vi "2. Color Classification.vi"() -> ()   [LabVIEW 2019]
doc: "c 2020 ReMiSYS All rights reserved."
panel:
  out "Colors 2":string[](array[string])
  out "Colors":string[](array[string])
  out "appended path":path
  out "Input Image":T1(plugin-control)
  in  "Stop (F)":bool caption="Stop"
  in  "Loop Delay (ms)":u32(slide)=1000 scale=0.0..1500.0
  # "c 2020 ReMiSYS All rights reserved."
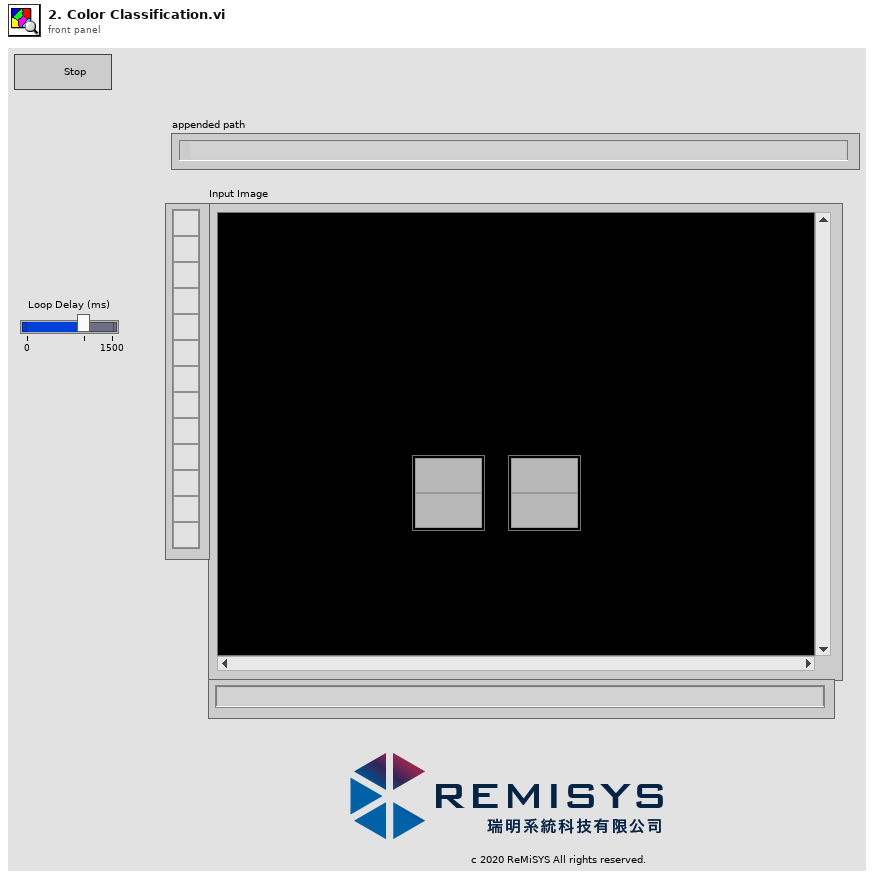
[diagram p1: front panel]
types:
  T1 = typedef "IMAQ Image.ctl" = refnum<image>
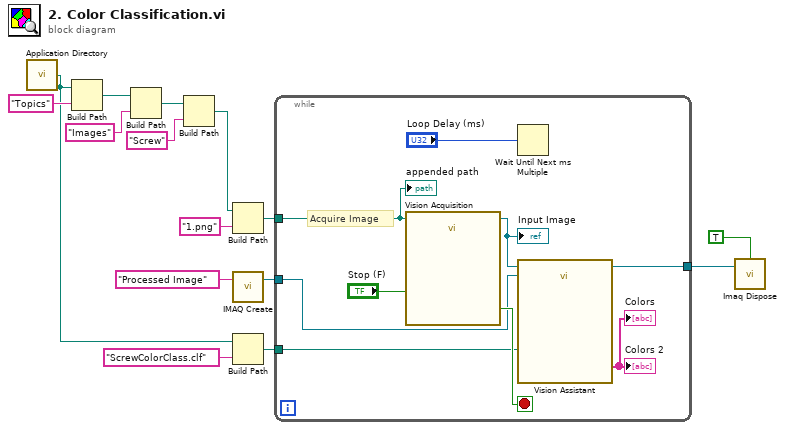
[diagram p0: block diagram]
diagram:
  n1 = call <vilib>:"Application Directory.vi"() -> ("Application Directory"=w1:path)
  n2 = Build Path(base path=w1, name or relative path="Topics") -> (appended path=w12:path)
  n3 = Build Path(base path=w12, name or relative path="Images") -> (appended path=w4:path)
  n4 = Build Path(base path=w4, name or relative path="Screw") -> (appended path=w5:path)
  n5 = Build Path(base path=w5, name or relative path="1.png") -> (appended path=w9:path)
  n6 = call "IMAQ Create"("Image Name"="Processed Image") -> ("New Image"=w15:T1)  [unwired: 3 in, 2 out]
  n7 = Build Path(base path=w1, name or relative path="ScrewColorClass.clf") -> (appended path=w2:path)
  n8 = while {
    tunnel: w15 -> [w20]
    tunnel: w9 -> [w21]
    tunnel: [w18] -> w8
    tunnel: w2 -> [w17]
    stop <- w24 stop-if-true
    # "Acquire Image"
    n9 = call "Vision Acquisition"("Image Path"=w21, "Stop (F)"="Stop (F)") -> ("Image Out"=w19:T1, "Stopped"=w24:bool)  [unwired: 1 in, 23 out]
    "Input Image" <- w19
    n10 = Wait Until Next ms Multiple(millisecond multiple="Loop Delay (ms)") -> ()  [unwired: 1 out]
    n11 = call "Vision Assistant"("Image In"=w19, "Image Dst"=w20, "File Path (Color Classification 1)"=w17) -> ("Image Out"=w18:T1, "Classes (Color Classification 1)"=→"Colors" →"Colors 2":string[])  [unwired: 22 in, 1 out]
    "appended path" <- w21
  }
  n12 = call "Imaq Dispose"("All Images? (No)"=TRUE, "Image"=w8) -> ()  [unwired: 4 in, 1 out]
